vi "Construct Controller.vi"(7 "UI.lvclass":refnum<class "UI.lvclass">, 8 "error in (no error)":errorcluster, 9 "Root Path":path, 10 "Configuration.lvlib:Configuration.lvclass":refnum<class "Configuration.lvclass">, 11 "Controller Actor.lvlib:Controller.lvclass":refnum<class "Controller.lvclass">) -> (0 "error out":errorcluster, 2 "Path to config file":path, 3 "Controller Actor.lvlib:Controller.lvclass 2":refnum<class "Controller.lvclass">)   [LabVIEW 2026, in "Controller Actor.lvlib" / "Controller.lvclass"]
uses:
  Controller.lvclass
  Controller.lvclass/Controller.ctl
  configuration/Configuration.lvclass
  <userlib>/_OpenG.lib/file/file.llb/File Exists - Scalar__ogtk.vi
  <userlib>/_OpenG.lib/file/file.llb/Valid Path - Traditional__ogtk.vi
  User Interface/UI.lvclass
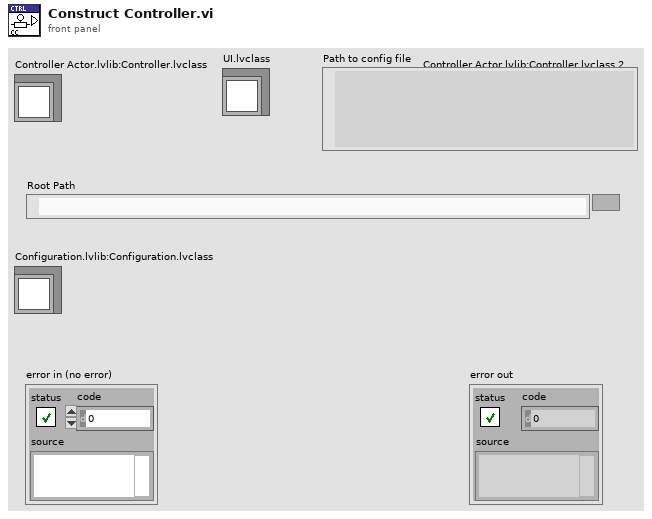
[diagram p1: front panel]
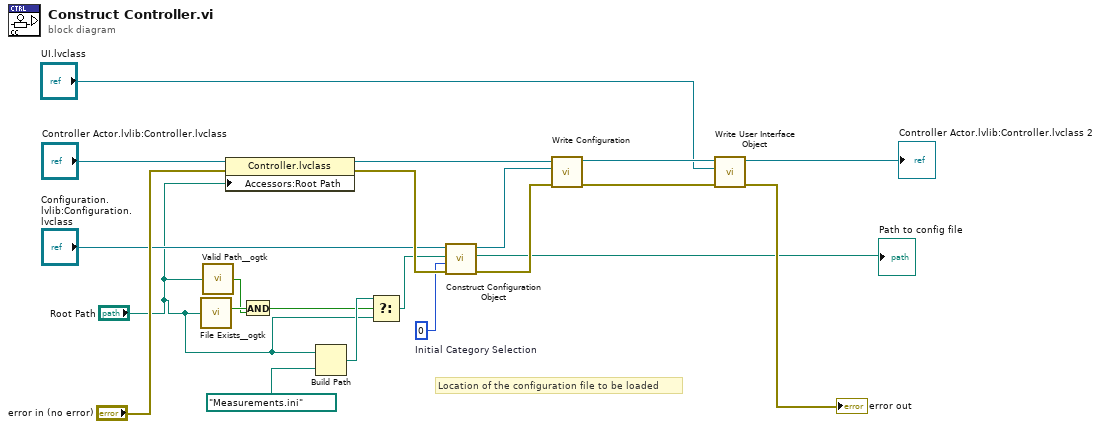
[diagram p0: block diagram]
diagram:
  w12 = 0  # Initial Category Selection
  # "Location of the configuration file to be loaded"
  n1 = call-poly <userlib>:"File Exists__ogtk.vi"("file path"="Root Path") -> ("is directory"=w4:bool)  [unwired: 6 in, 1 out]
  n2 = call-poly <userlib>:"Valid Path__ogtk.vi"("path"="Root Path") -> ("valid"=w1:bool)
  n3 = property class="Controller.lvclass"(reference="Controller Actor.lvlib:Controller.lvclass", error in="error in (no error)", "Accessors:Root Path"="Root Path") -> (reference out=w15:refnum<class "Controller.lvclass">, error out=w14:errorcluster)
  n4 = And(x=w4, y=w1) -> (x .and. y?=w3:bool)
  n5 = Build Path(base path="Root Path", name or relative path=path "Measurements.ini" ("VI Path")) -> (appended path=w6:path)
  n6 = Select(t=w6, s=w3, f="Root Path") -> (s? t:f=w5:path)
  n7 = call "Construct Configuration Object.vi"("error in (no error)"=w14, "Initial Category Selection"=w12, "Configuration File Path"=w5, "Configuration in"="Configuration.lvlib:Configuration.lvclass") -> ("error out"=w17:errorcluster, "Path to config file"=→"Path to config file":path, "Configuration out"=w18:refnum<class "Configuration.lvclass">)  [unwired: 4 in, 1 out]
  n8 = call "Write Configuration.vi"("error in (no error)"=w17, "Configuration.lvlib:Configuration.lvclass"=w18, "Controller in"=w15) -> ("error out"=w19:errorcluster, "Controller out"=w20:refnum<class "Controller.lvclass">)  [unwired: 7 in]
  n9 = call "Write User Interface Object.vi"("error in (no error)"=w19, "UI.lvclass"="UI.lvclass", "UI Controller in"=w20) -> ("error out"=→"error out":errorcluster, "UI Controller out"=→"Controller Actor.lvlib:Controller.lvclass 2":refnum<class "Controller.lvclass">)  [unwired: 7 in]
